vi "prac2-1.vi"() -> ()   [LabVIEW 2014]
panel:
  in  "L2":dbl
  in  "L1":dbl
  in  "Angulo 2":dbl(knob)
  in  "Angulo 1":dbl(knob)
  out "XY Graph":cluster{dbl[], dbl[]}(graph)
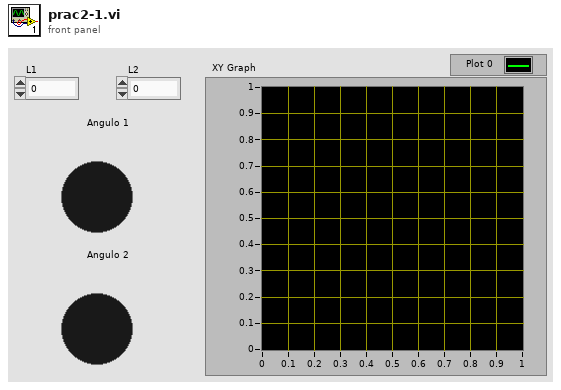
[diagram p1: front panel]
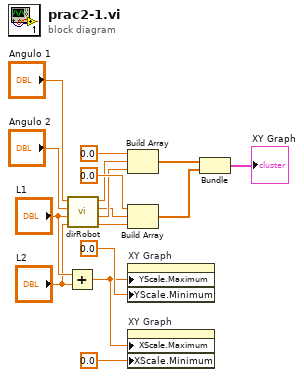
[diagram p0: block diagram]
diagram:
  n1 = Add(x="L1", y="L2") -> (x+y=w3:dbl)
  n2 = call "dirRobot.vi"("L2"="L2", "L1"="L1", "Angulo 2"="Angulo 2", "Angulo 1"="Angulo 1") -> ("y"=w11:dbl, "x"=w13:dbl, "y1"=w12:dbl, "x1"=w14:dbl)
  n3 = Build Array "Build Array"(0.0 ("element"), w14, w13) -> (w10:dbl[])
  n4 = Build Array "Build Array"(0.0 ("element"), w12, w11) -> (w9:dbl[])
  n5 = property on="XY Graph" class="XYGraph (strict)"("YScale.Maximum"=w3, "YScale.Minimum"=0.0 ("Y Scale.Range:Minimum")) -> ()  [unwired: 2 in, 2 out]
  n6 = property on="XY Graph" class="XYGraph (strict)"("XScale.Maximum"=w3, "XScale.Minimum"=0.0 ("X Scale.Range:Minimum")) -> ()  [unwired: 2 in, 2 out]
  n7 = Bundle "Bundle"(w10, w9) -> (→"XY Graph":cluster{dbl[], dbl[]})  [unwired: 1 in]
